vi "write_serial_cmd_Nchan.vi"(5 "which manipulator":T1(ring), 6 "arg 2":i32, 8 "error in":errorcluster, 9 "arg 1":dbl, 10 "pressure command":T2, 11 "Pressure Box COM":refnum<visa-resource-name>) -> (0 "error out":errorcluster, 3 "Pressure Box COM out":refnum<visa-resource-name>)   [LabVIEW 2019]
uses:
  controls/proportionAir_cmds.ctl
  <vilib>/Instr/_visa.llb/VISA Flush IO Buffer Mask.ctl
panel:
  out "Response":string
  # "PROPORTIONAIR REGULATOR"
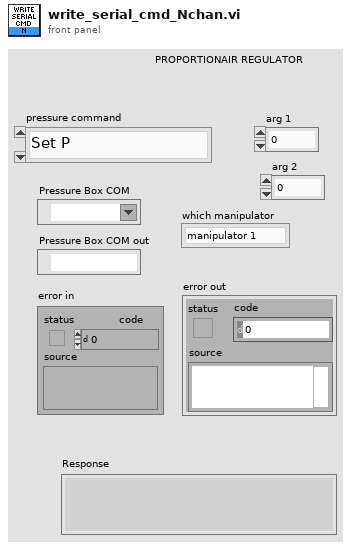
[diagram p1: front panel]
types:
  T1 = enum16{"manipulator 1", "manipulator 2", "manipulator 3", "manipulator 4"}
  T2 = typedef "proportionAir_cmds.ctl" = enum16{"Set P", "Switch to Atm", "Switch to Regulator", "Pulse", "WC"}
  T3 = typedef "VISA Flush IO Buffer Mask.ctl" = u16
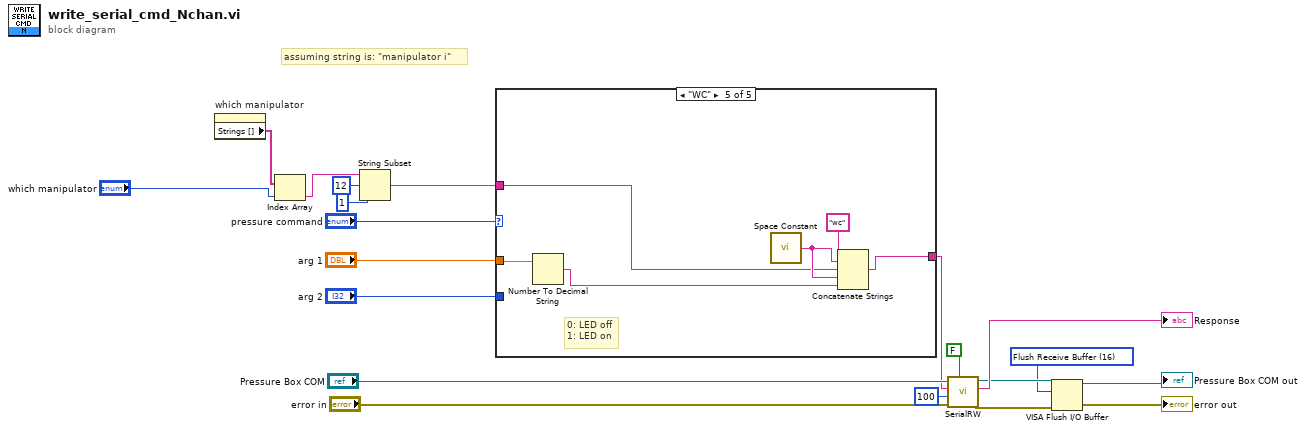
[diagram p0: block diagram]
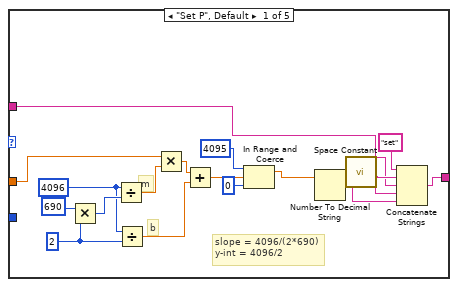
[diagram p2: hidden frame]
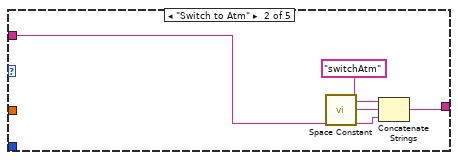
[diagram p3: hidden frame]
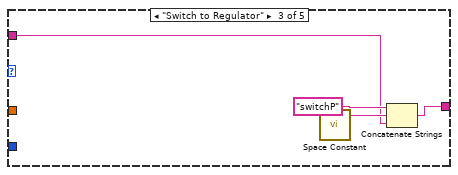
[diagram p4: hidden frame]
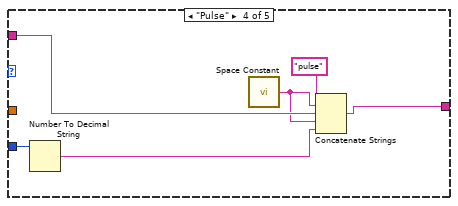
[diagram p5: hidden frame]
diagram:
  w7 = T3 16 items=["Flush Receive Buffer"=16, "Write Transmit Buffer to Device"=32, "Flush Receive Buffer (No I/O)"=64, "Flush Transmit Buffer"=128] ("Mask")
  # "assuming string is: \"manipulator i\""
  n1 = property on="which manipulator" class="Enum (strict)"() -> ("Strings []"=w6:string[])  [unwired: 2 in, 2 out]
  n2 = Index Array(array=w6, index="which manipulator") -> (element=w4:string)
  n3 = String Subset(string=w4, offset (0)=12, length (rest)=1 ("length (rest)")) -> (substring=w1:string)
  n4 = case shown="\"WC\"" "pressure command" {
    tunnel: "arg 1" -> [w24 _ _ _ w54]
    tunnel: [w36 w38 w42 w49 w52] -> w14
    tunnel: "arg 2" -> [_ _ _ w50 _]
    tunnel: w1 -> [w21 w39 w43 w48 w55]
    frame "Set P", Default {
      w32 = 2 ("y")
      w33 = 4096
      # "b"
      # "m"
      # "slope = 4096/(2*690)\ny-int = 4096/2"
      n5 = Multiply(x=690, y=w32) -> (x*y=w34:i32)
      n6 = Divide(x=w33, y=w34) -> (x/y=w31:dbl)
      n7 = Divide(x=w33, y=w32) -> (x/y=w30:dbl)
      n8 = Multiply(x=w24, y=w31) -> (x*y=w29:dbl)
      n9 = Add(x=w29, y=w30) -> (x+y=w28:dbl)
      n10 = In Range and Coerce(upper limit=4095, x=w28, lower limit=0) -> (coerced(x)=w25:dbl)  [unwired: 1 out]
      n11 = Number To Decimal String(number=w25) -> (decimal integer string=w22:string)  [unwired: 1 in]
      n12 = call <vilib>:"Space Constant.vi"() -> ("String"=w23:string)
      n13 = Concatenate Strings("set" ("string"), w23, w21, w23, w22) -> (w36:string)
    }
    frame "Switch to Atm" {
      n14 = call <vilib>:"Space Constant.vi"() -> ("String"=w40:string)
      n15 = Concatenate Strings("switchAtm", w40, w39) -> (w38:string)
    }
    frame "Switch to Regulator" {
      n16 = call <vilib>:"Space Constant.vi"() -> ("String"=w44:string)
      n17 = Concatenate Strings("switchP", w44, w43) -> (w42:string)
    }
    frame "Pulse" {
      n18 = Number To Decimal String(number=w50) -> (decimal integer string=w46:string)  [unwired: 1 in]
      n19 = call <vilib>:"Space Constant.vi"() -> ("String"=w47:string)
      n20 = Concatenate Strings("pulse" ("string"), w47, w48, w47, w46) -> (w49:string)
    }
    frame "WC" {
      # "0: LED off\n1: LED on"
      n21 = Number To Decimal String(number=w54) -> (decimal integer string=w53:string)  [unwired: 1 in]
      n22 = call <vilib>:"Space Constant.vi"() -> ("String"=w56:string)
      n23 = Concatenate Strings("wc" ("string"), w56, w55, w56, w53) -> (w52:string)
    }
  }
  n24 = call "SerialRW.vi"("Query?"=FALSE, "error in (no error)"="error in", "Delay (ms)"=u32 100, "Command"=w14, "VISA handle"="Pressure Box COM") -> ("error out"=w10:errorcluster, "Response"=→"Response":string, "Dup. VISA handle"=w11:refnum<visa-resource-name>)  [unwired: 1 in, 1 out]
  n25 = VISA Flush I/O Buffer(VISA resource name=w11, mask (16)=w7, error in (no error)=w10) -> (VISA resource name out=→"Pressure Box COM out":refnum<visa-resource-name>, error out=→"error out":errorcluster)
